vi "Get Currents.vi"(11 "AER in":refnum<class "AER.lvclass">) -> (1 "No N":i32[](array[numeric]), 2 "Currents":dbl[](array[numeric]), 3 "AER out":refnum<class "AER.lvclass">)   [LabVIEW 2013, in "AER.lvclass"]
uses:
  AER.lvclass
  AER.lvclass/AER.ctl
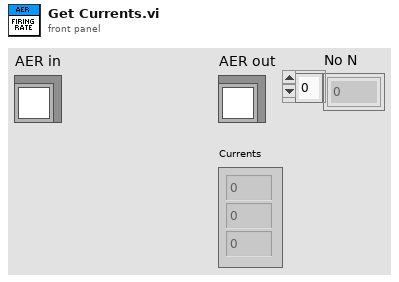
[diagram p1: front panel]
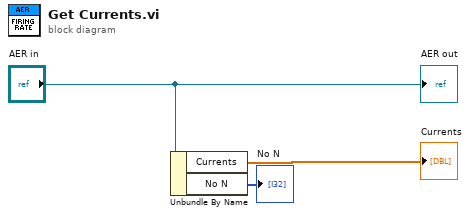
[diagram p0: block diagram]
diagram:
  n1 = Unbundle By Name("AER in") -> ("Currents"=→"Currents":dbl[], "No N"=→"No N":i32[])
  "AER out" <- "AER in"
